vi "Resolve VI Path.vi"(8 "error in (no error)":errorcluster, 10 "Alt Dir (\"\")":path, 11 "Qualified Name (lvlibp|lvlib[:vi])":string) -> (0 "error out":errorcluster, 3 "VI Path":path)   [LabVIEW 2022 SP3, in "Core.lvlib"]
uses:
  Core.lvlib
  <vilib>/Utility/LVLibp/NI_PackedLibraryUtility.lvlib
  Demo.vi
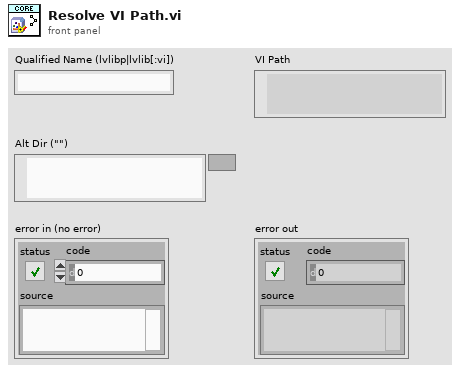
[diagram p1: front panel]
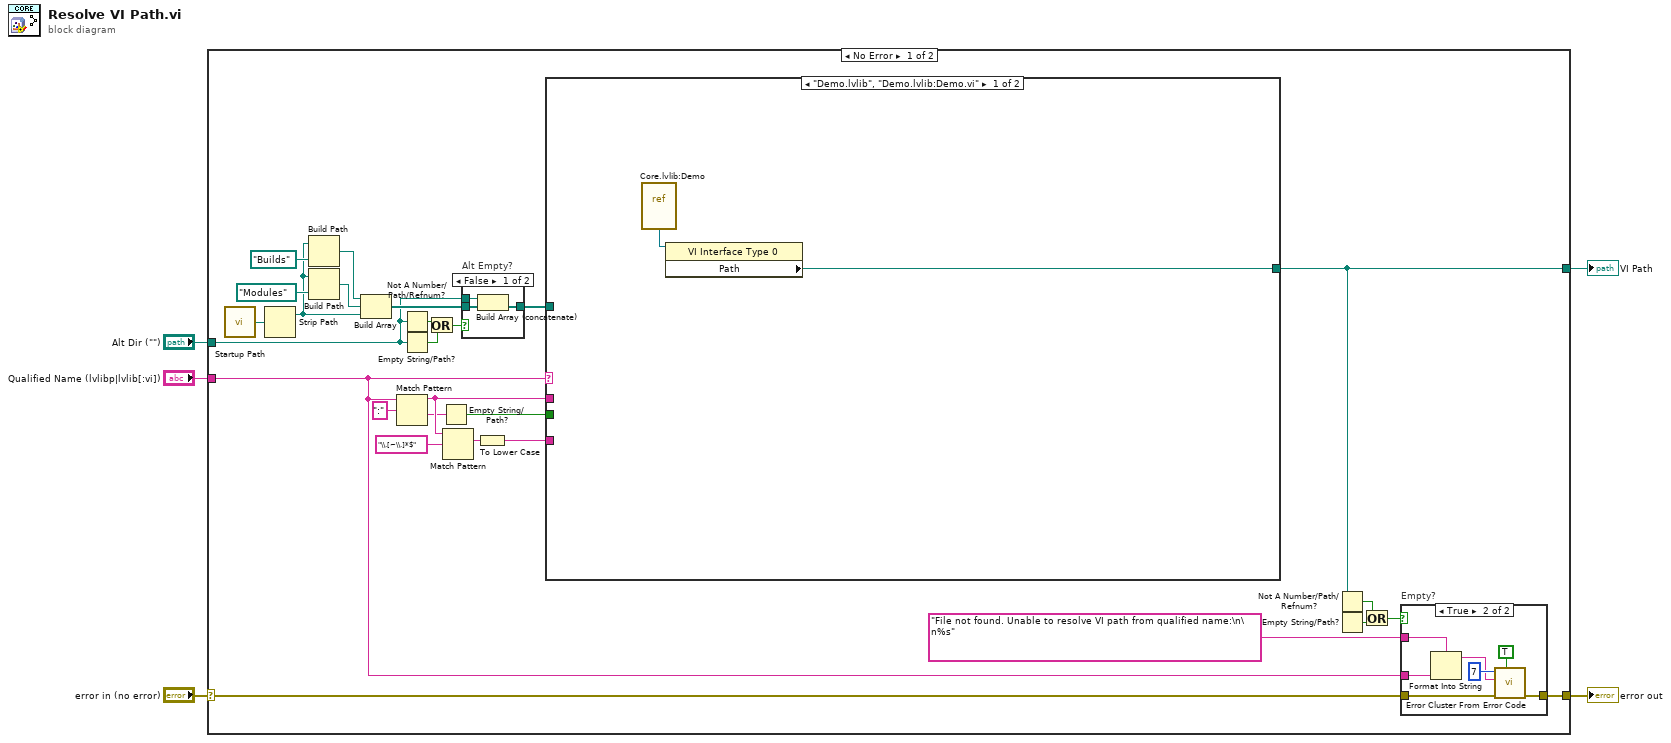
[diagram p0: block diagram]
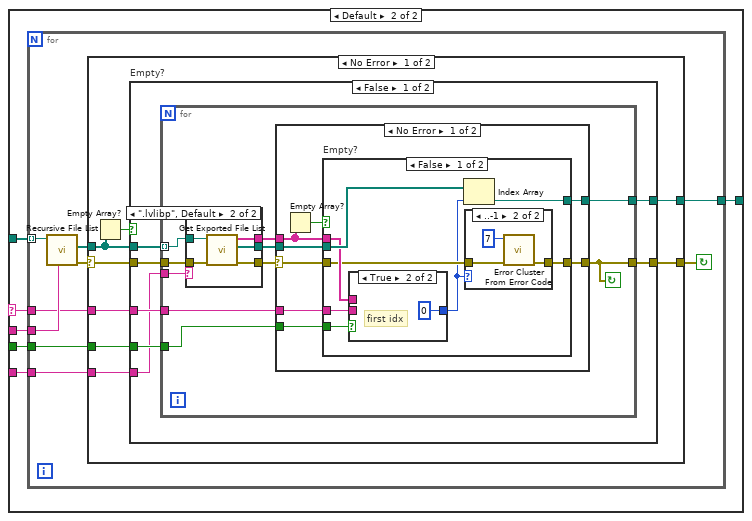
[diagram p2: hidden frame]
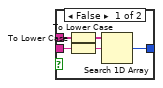
[diagram p5: hidden frame]
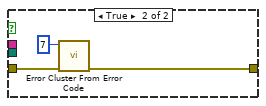
[diagram p6: hidden frame]
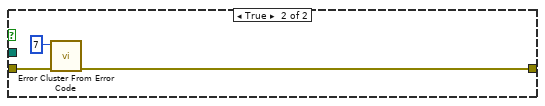
[diagram p8: hidden frame]
diagram:
  n1 = case shown="No Error" "error in (no error)" {
    selector: "error in (no error)" -> [w13 w127]
    tunnel: "Qualified Name (lvlibp|lvlib[:vi])" -> [w8 _]
    tunnel: [w12 w127] -> w3
    tunnel: "Alt Dir (\"\")" -> [w22 _]
    tunnel: [w9 _] -> w1
    frame No Error {
      n2 = call "Startup Path.vi"() -> ("Startup.ini"=w28:path)
      n3 = Strip Path(path=w28) -> (stripped path=w25:path)  [unwired: 1 out]
      n4 = Build Path(base path=w25, name or relative path=path "Builds") -> (appended path=w24:path)
      n5 = Build Path(base path=w25, name or relative path=path "Modules") -> (appended path=w17:path)
      n6 = Build Array(w24, w17, w25) -> (w23:path[])
      n7 = Match Pattern(string=w8, regular expression=":") -> (before substring=w30:string, after substring=w15:string)  [unwired: 1 in, 2 out]
      n8 = Not A Number/Path/Refnum?(number/path/refnum=w22) -> (NaN/Path/Refnum?=w20:bool)
      n9 = Empty String/Path?(string/path=w22) -> (empty?=w21:bool)
      n10 = Or(x=w20, y=w21) -> (x .or. y?=w19:bool)
      n11 = Empty String/Path?(string/path=w15) -> (empty?=w14:bool)
      n12 = Match Pattern(string=w30, regular expression="\\.[~\\.]*$") -> (match substring=w29:string)  [unwired: 4 out]
      n13 = case "Alt Empty?" shown="False" w19 {
        tunnel: w23 -> [w117 w118]
        tunnel: w22 -> [w116 _]
        tunnel: [w115 w118] -> w18
        frame False {
          n14 = Build Array (concatenate)(w116, w117) -> (w115:path[])
        }
        frame True {
        }
      }
      n15 = To Lower Case(string=w29) -> (all lower case string=w16:string)
      n16 = case shown="\"Demo.lvlib\", \"Demo.lvlib:Demo.vi\"" w8 {
        selector: w8 -> [_ w35]
        tunnel: w30 -> [_ w40]
        tunnel: w18 -> [_ w39]
        tunnel: w16 -> [_ w38]
        tunnel: w14 -> [_ w37]
        tunnel: [w34 w36] -> w9
        frame "Demo.lvlib", "Demo.lvlib:Demo.vi" {
          n17 = vi-ref "Core.lvlib:Demo.vi"() -> (w33:refnum<vi>)
          n18 = property class="VI Interface Type 0"(reference=w33) -> ("Path"=w34:path)  [unwired: 1 in, 2 out]
        }
        frame Default {
          n19 = for {
            tunnel: w40 -> [w49]
            tunnel: w35 -> [w47]
            tunnel: w39 -> [w46] mode=indexing
            tunnel: w38 -> [w45]
            tunnel: w37 -> [w43]
            tunnel: [w42] -> w36
            stop <- w41 continue-if-true
            n20 = call <vilib>:"Recursive File List.vi"("pattern"=w49, "Folder Path"=w46) -> ("error out"=w48:errorcluster, "All Files in Dir"=w44:path[])  [unwired: 5 in, 3 out]
            n21 = case shown="No Error" w48 {
              selector: w48 -> [w57 w114]
              tunnel: w47 -> [w56 _]
              tunnel: w45 -> [w55 _]
              tunnel: w44 -> [w54 _]
              tunnel: w43 -> [w52 _]
              tunnel: [w51 _] -> w42
              tunnel: [w50 w114] -> w41
              frame No Error {
                n22 = Empty Array?(array=w54) -> (empty?=w53:bool)
                n23 = case "Empty?" shown="False" w53 {
                  tunnel: w54 -> [w58 _]
                  tunnel: w57 -> [w64 w113]
                  tunnel: [w63 w112] -> w50
                  tunnel: w56 -> [w62 _]
                  tunnel: w55 -> [w59 _]
                  tunnel: w52 -> [w61 _]
                  tunnel: [w60 _] -> w51
                  frame False {
                    n24 = for {
                      tunnel: w62 -> [w73]
                      tunnel: w61 -> [w72]
                      tunnel: [w71] -> w60
                      tunnel: w59 -> [w67]
                      tunnel: w64 -> [w74]
                      tunnel: [w65] -> w63
                      tunnel: w58 -> [w66] mode=indexing
                      stop <- w65 continue-if-true
                      n25 = case shown="\".lvlibp\", Default" w67 {
                        tunnel: w74 -> [w75 w80]
                        tunnel: [_ w79] -> w70
                        tunnel: [_ w78] -> w69
                        tunnel: [w75 w77] -> w68
                        tunnel: w66 -> [_ w76]
                        frame ".lvlib" {
                        }
                        frame ".lvlibp", Default {
                          n26 = call <vilib>:"Get Exported File List.vi"("error in (no error)"=w80, "packed library path"=w76) -> ("error out"=w77:errorcluster, "paths"=w79:path[], "qualified names"=w78:string[])  [unwired: 7 in]
                        }
                      }
                      n27 = case shown="No Error" w68 {
                        selector: w68 -> [w82 w110]
                        tunnel: w70 -> [w88 _]
                        tunnel: w73 -> [w87 _]
                        tunnel: w69 -> [w85 _]
                        tunnel: [w86 _] -> w71
                        tunnel: [w83 w110] -> w65
                        tunnel: w72 -> [w81 _]
                        frame No Error {
                          n28 = Empty Array?(array=w85) -> (empty?=w84:bool)
                          n29 = case "Empty?" shown="False" w84 {
                            tunnel: w88 -> [w96 _]
                            tunnel: w87 -> [w95 _]
                            tunnel: [w94 _] -> w86
                            tunnel: w85 -> [w93 _]
                            tunnel: [w90 w108] -> w83
                            tunnel: w82 -> [w92 w107]
                            tunnel: w81 -> [w91 _]
                            frame False {
                              n30 = case shown="True" w91 {
                                tunnel: w95 -> [w105 _]
                                tunnel: [w102 0 ("index of element")] -> w89
                                tunnel: w93 -> [w101 _]
                                frame False {
                                n31 = To Lower Case(string=w101) -> (all lower case string=w103:string[])
                                n32 = To Lower Case(string=w105) -> (all lower case string=w104:string)
                                n33 = Search 1D Array(1D array=w103, element=w104) -> (index of element=w102:i32)  [unwired: 1 in]
                                }
                                frame True {
                                # "first idx"
                                }
                              }
                              n34 = Index Array(array=w96, index=w89) -> (element=w94:path)
                              n35 = case shown="..-1" w89 {
                                tunnel: w92 -> [w97 w100]
                                tunnel: [w97 w99] -> w90
                                frame 0.. {
                                }
                                frame ..-1 {
                                n36 = call <vilib>:"Error Cluster From Error Code.vi"("error in (no error)"=w100, "error code (0)"=7) -> ("error out"=w99:errorcluster)  [unwired: 7 in]
                                }
                              }
                            }
                            frame True {
                              n37 = call <vilib>:"Error Cluster From Error Code.vi"("error in (no error)"=w107, "error code (0)"=7) -> ("error out"=w108:errorcluster)  [unwired: 7 in]
                            }
                          }
                        }
                        frame Error {
                        }
                      }
                    }
                  }
                  frame True {
                    n38 = call <vilib>:"Error Cluster From Error Code.vi"("error in (no error)"=w113, "error code (0)"=7) -> ("error out"=w112:errorcluster)  [unwired: 7 in]
                  }
                }
              }
              frame Error {
              }
            }
          }
        }
      }
      n39 = Not A Number/Path/Refnum?(number/path/refnum=w9) -> (NaN/Path/Refnum?=w11:bool)
      n40 = Empty String/Path?(string/path=w9) -> (empty?=w10:bool)
      n41 = Or(x=w11, y=w10) -> (x .or. y?=w6:bool)
      n42 = case "Empty?" shown="True" w6 {
        tunnel: w13 -> [w119 w126]
        tunnel: [w119 w125] -> w12
        tunnel: w8 -> [_ w122]
        tunnel: "File not found. Unable to resolve VI path from qualified name:\n\n%s" ("format string") -> [_ w121]
        frame False {
        }
        frame True {
          n43 = Format Into String(format string=w121, w122) -> (resulting string=w120:string)  [unwired: 2 in, 1 out]
          n44 = call <vilib>:"Error Cluster From Error Code.vi"("show call chain? (False)"=TRUE, "error in (no error)"=w126, "error message (\"\")"=w120, "error code (0)"=7) -> ("error out"=w125:errorcluster)  [unwired: 5 in]
        }
      }
    }
    frame Error {
    }
  }
  "error out" <- w3
  "VI Path" <- w1
